vi "gold--constant.vi"() -> (1 "Gold":u32)   [LabVIEW 2018, in "Resistor Band Colors.lvlib"]
uses:
  Resistor Band Colors.lvlib
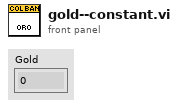
[diagram p1: front panel]
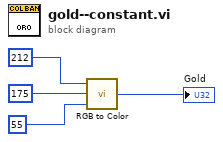
[diagram p0: block diagram]
diagram:
  n1 = call <vilib>:"RGB to Color.vi"("B"=u8 55 ("R"), "G"=u8 175 ("R"), "R"=u8 212) -> ("Color"=→"Gold":u32)
